vi "Write Interval (ms).vi"(8 "error in (no error)":errorcluster, 10 "Interval (ms)":dbl, 11 "Synchronization Device in":refnum<class "Synchronization Device.lvclass">) -> (0 "error out":errorcluster, 3 "Synchronization Device out":refnum<class "Synchronization Device.lvclass">)   [LabVIEW 2018]
uses:
  Synchronization Device.lvclass
  C:/LVCUR/flash-gordon/Hardware/Device/Device.lvclass
  C:/Program Files/National Instruments/LabVIEW 2018/vi.lib/ActorFramework/Actor/Actor.lvclass
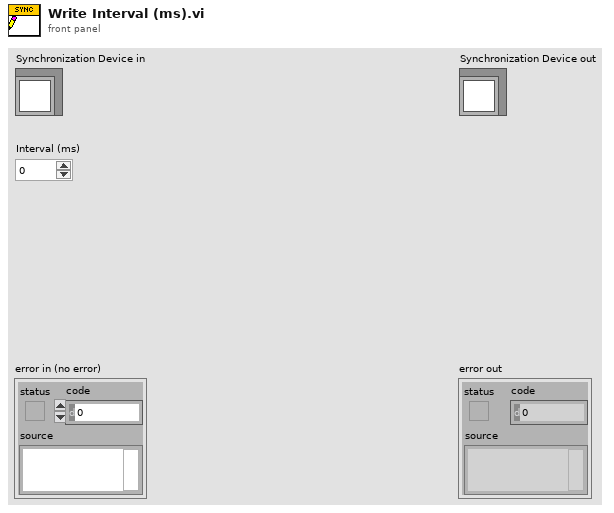
[diagram p1: front panel]
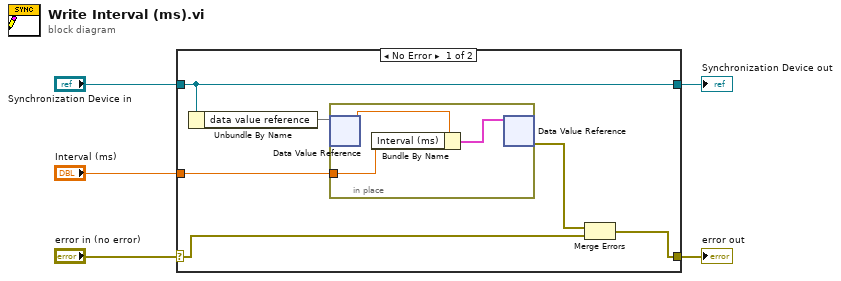
[diagram p0: block diagram]
diagram:
  n1 = case shown="No Error" "error in (no error)" {
    selector: "error in (no error)" -> [w7 w15]
    tunnel: [w8 w15] -> w4
    tunnel: [w9 w16] -> w2
    tunnel: "Synchronization Device in" -> [w9 w16]
    tunnel: "Interval (ms)" -> [w10 _]
    frame No Error {
      n2 = Unbundle By Name(w9) -> ("data value reference"=w11)
      n3 = in-place {
        in-place-border: w10 -> [w14]
        n4 = in-place-dvr #1(w11) -> (w13:dbl)  [unwired: 1 out]
        n5 = Bundle By Name(cluster=w13, "Interval (ms)"=w14) -> (w12:cluster{})
        n6 = in-place-dvr #1(w12) -> (w6:errorcluster)  [unwired: 1 out]
      }
      n7 = Merge Errors(w6, w7) -> (w8:errorcluster)
    }
    frame Error {
    }
  }
  "error out" <- w4
  "Synchronization Device out" <- w2
